vi "VAT_valve_adjust_setpoint.vi"(0 "VAT Valve COM port":refnum<visa-resource-name>, 1 "Flow":dbl, 3 "Pressure":dbl, 5 "Operating Mode":u16(ring) items=["Pressure", "Flow"], 9 "Unit":string, 11 "error in (no error)":errorcluster) -> (4 "VAT Valve COM port out":refnum<visa-resource-name>, 15 "error out":errorcluster)   [LabVIEW 2019]
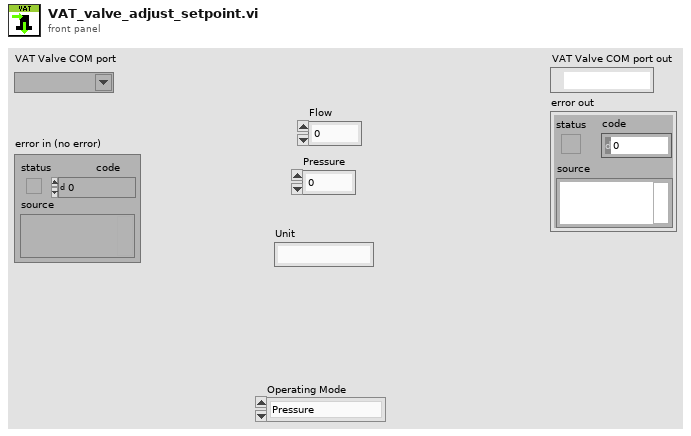
[diagram p1: front panel]
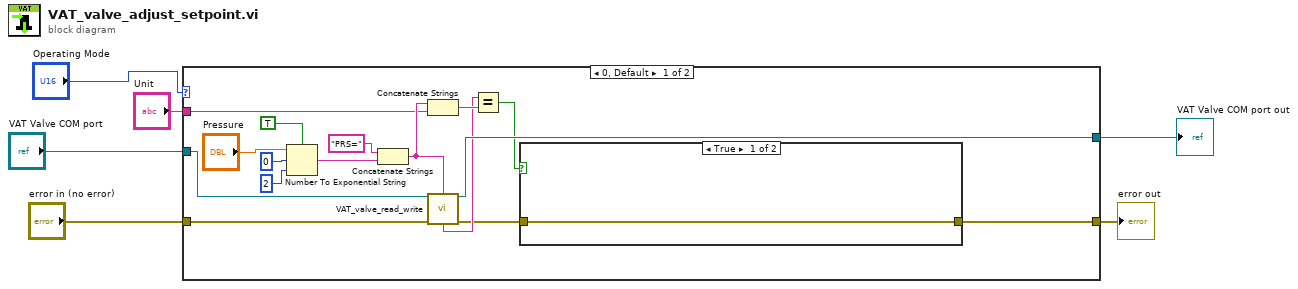
[diagram p0: block diagram]
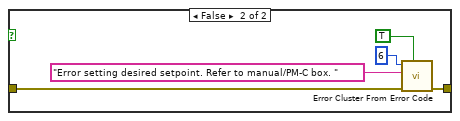
[diagram p2: hidden frame]
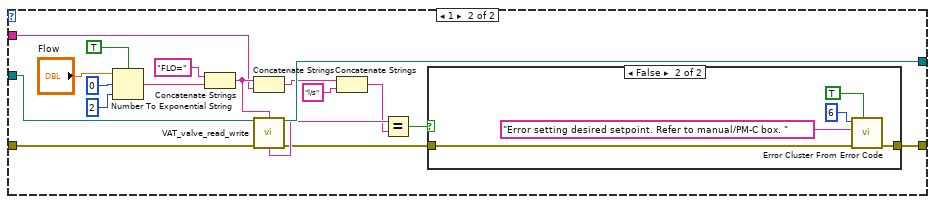
[diagram p3: hidden frame]
diagram:
  n1 = case shown="0, Default" "Operating Mode" {
    tunnel: "VAT Valve COM port" -> [w22 w46]
    tunnel: "error in (no error)" -> [w21 w45]
    tunnel: [w14 w38] -> w3
    tunnel: "Unit" -> [w12 w36]
    tunnel: [w7 w29] -> w1
    frame 0, Default {
      n2 = Number To Exponential String(number="Pressure", precision (6)=i16 2, 1:TRUE ("use system decimal point (T)"), 3:i16 0 ("width (-)")) -> (E-format string=w15:string)
      n3 = Concatenate Strings("PRS=" ("string"), w15) -> (w13:string)
      n4 = Concatenate Strings(w13, w12) -> (w11:string)
      n5 = call "VAT_valve_read_write.vi"("VAT Valve COM port"=w22, "Write String"=w13, "error in (no error)"=w21) -> ("VAT Valve COM port out"=w14:refnum<visa-resource-name>, "Read String"=w10:string, "error out"=w8:errorcluster)  [unwired: 10 in]
      n6 = Equal?(x=w10, y=w11) -> (x = y?=w9:bool)
      n7 = case shown="True" w9 {
        tunnel: w8 -> [w23 w28]
        tunnel: [w23 w24] -> w7
        frame True {
        }
        frame False {
          n8 = call <vilib>:"Error Cluster From Error Code.vi"("show call chain? (False)"=TRUE, "error in (no error)"=w28, "error message (\"\")"="Error setting desired setpoint. Refer to manual/PM-C box. " ("error message (\"\")"), "error code (0)"=6) -> ("error out"=w24:errorcluster)  [unwired: 5 in]
        }
      }
    }
    frame 1 {
      n9 = Number To Exponential String(number="Flow", precision (6)=i16 2, 1:TRUE ("use system decimal point (T)"), 3:i16 0 ("width (-)")) -> (E-format string=w39:string)
      n10 = Concatenate Strings("FLO=" ("string"), w39) -> (w37:string)
      n11 = Concatenate Strings(w37, w36) -> (w32:string)
      n12 = call "VAT_valve_read_write.vi"("VAT Valve COM port"=w46, "Write String"=w37, "error in (no error)"=w45) -> ("VAT Valve COM port out"=w38:refnum<visa-resource-name>, "Read String"=w35:string, "error out"=w33:errorcluster)  [unwired: 10 in]
      n13 = Concatenate Strings(w32, "l/s" ("string")) -> (w30:string)
      n14 = Equal?(x=w35, y=w30) -> (x = y?=w34:bool)
      n15 = case shown="False" w34 {
        tunnel: w33 -> [w47 w52]
        tunnel: [w47 w48] -> w29
        frame True {
        }
        frame False {
          n16 = call <vilib>:"Error Cluster From Error Code.vi"("show call chain? (False)"=TRUE, "error in (no error)"=w52, "error message (\"\")"="Error setting desired setpoint. Refer to manual/PM-C box. " ("error message (\"\")"), "error code (0)"=6) -> ("error out"=w48:errorcluster)  [unwired: 5 in]
        }
      }
    }
  }
  "VAT Valve COM port out" <- w3
  "error out" <- w1
